vi "Set Property Value.vi"(8 "error in":errorcluster, 10 "Property Type":T1, 11 "Property Type Node":refnum<k20>) -> (0 "error out":errorcluster, 2 "Property Value":variant, 3 "Property Type Node":refnum<k20>)   [LabVIEW 2024, in "Config File Parser.lvlib" / "Property.lvclass"]
uses:
  Property.lvclass
  Property Type.ctl
  DependentFile.ctl
  <vilib>/xml/Close Reference(Node).vi
  Property.lvclass/Property.ctl
  <resource>/objmgr/DOMUserDefRef.rc
  <vilib>/xml/NI_XML.lvlib
  Config File Parser.lvlib
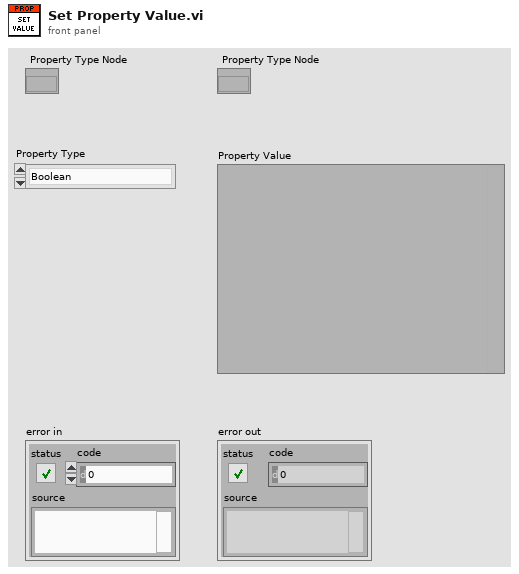
[diagram p1: front panel]
types:
  T1 = typedef "Config File Parser.lvlib/Property.lvclass/Property Type.ctl" = enum16{"Boolean", "Double", "String", "Path", "Dictionary", "DependentFile", "I16", "I32", "I64", "U16", "U32", "U64", "BooleanArray", "DoubleArray", "StringArray", "I16Array", "I32Array", "I64Array", "U16Array", "U32Array", "U64Array", "Variant"}
  T2 = typedef "Config File Parser.lvlib/Property.lvclass/DependentFile.ctl" = cluster{"Path":path, "Version":string, "RTDestination":path, "ForceDownload":bool, "SupportedTarget":string, "MD5":string, " Type":string}
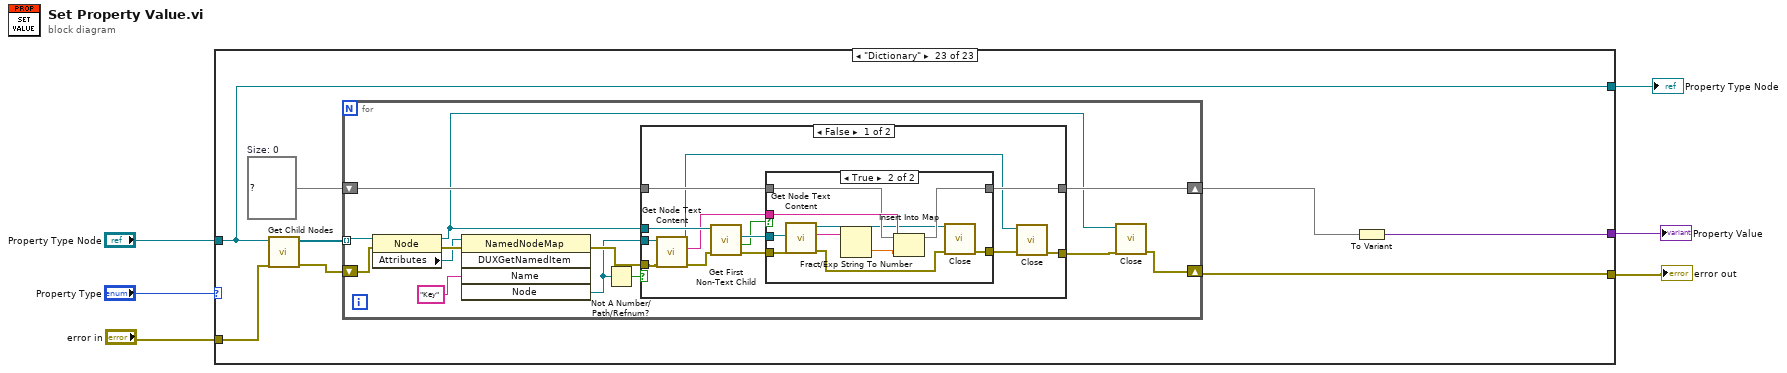
[diagram p0: block diagram]
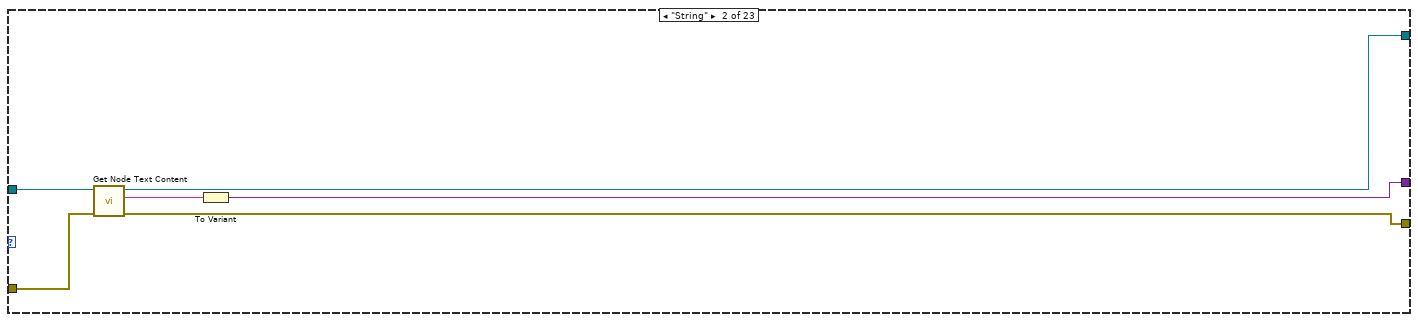
[diagram p3: hidden frame]
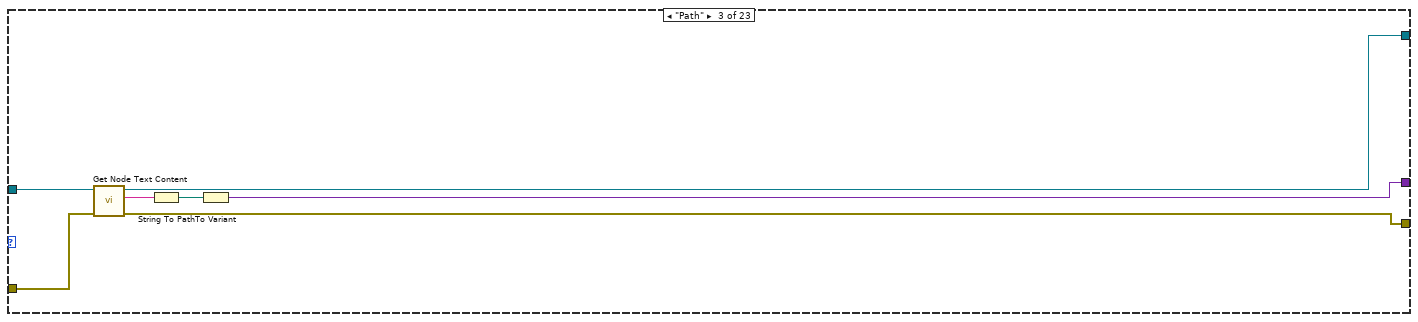
[diagram p4: hidden frame]
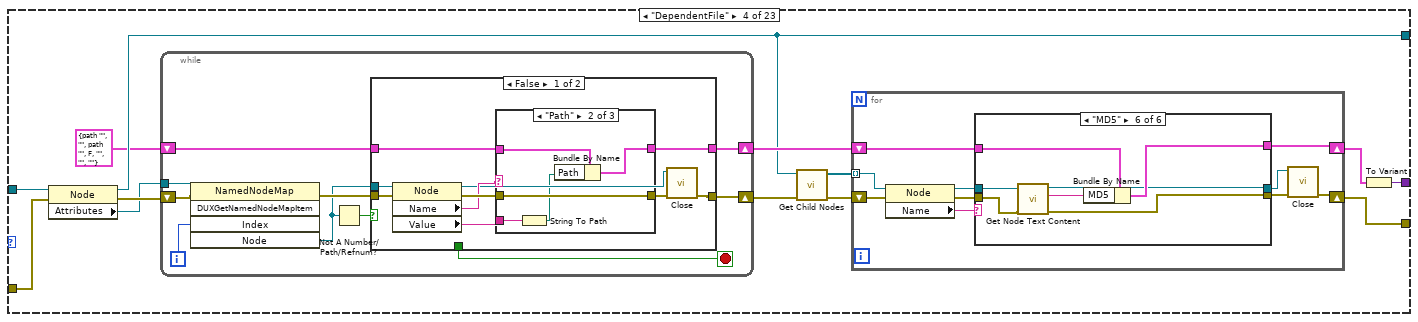
[diagram p5: hidden frame]
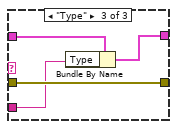
[diagram p7: hidden frame]
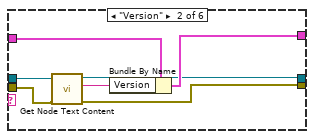
[diagram p10: hidden frame]
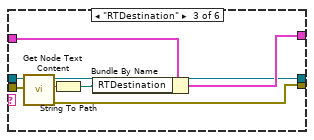
[diagram p11: hidden frame]
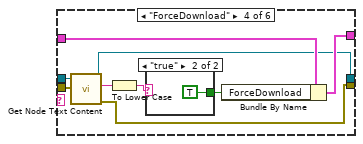
[diagram p12: hidden frame]
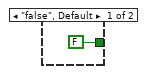
[diagram p13: hidden frame]
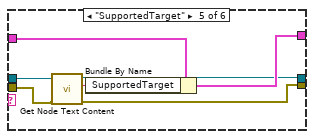
[diagram p14: hidden frame]
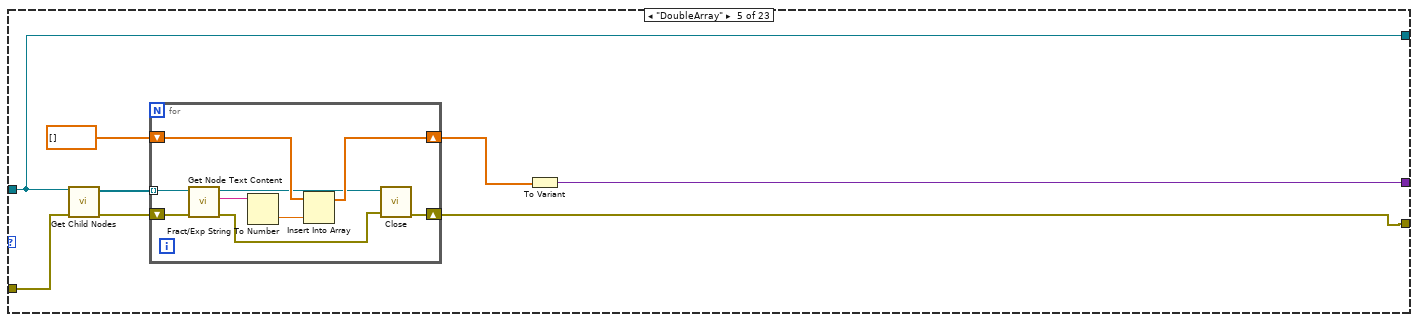
[diagram p15: hidden frame]
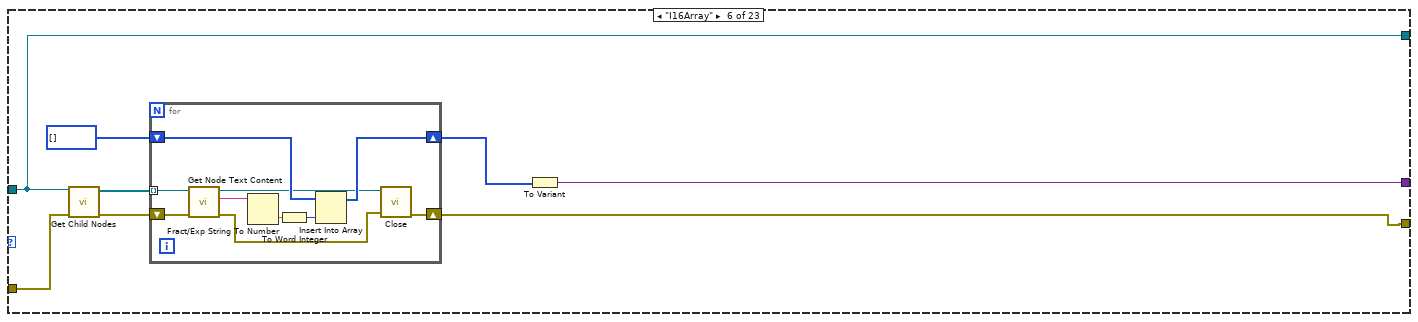
[diagram p16: hidden frame]
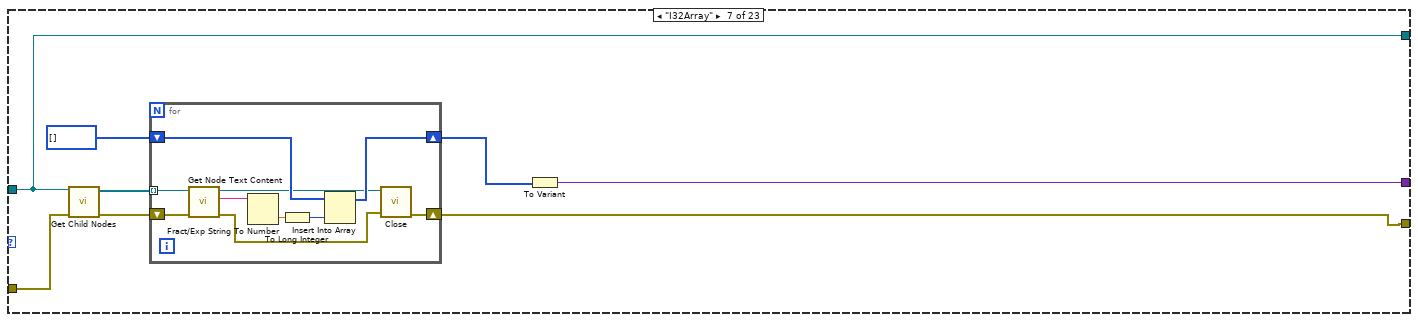
[diagram p17: hidden frame]
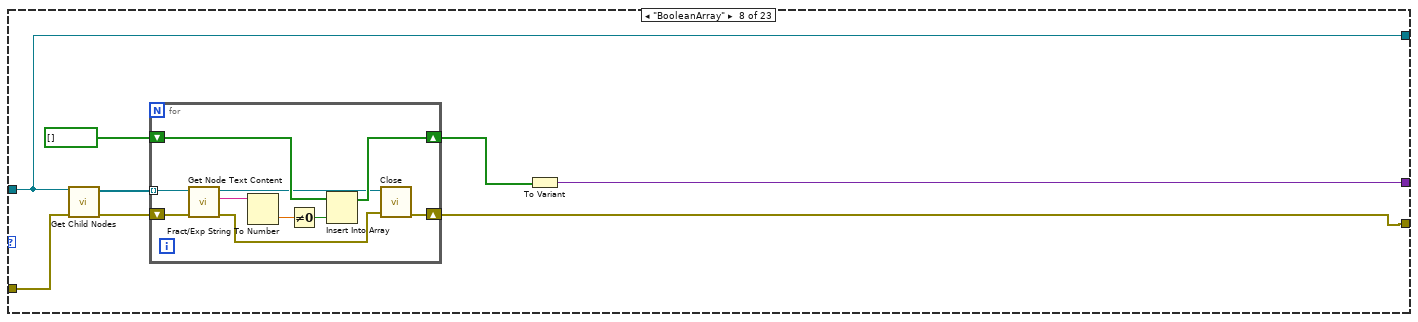
[diagram p18: hidden frame]
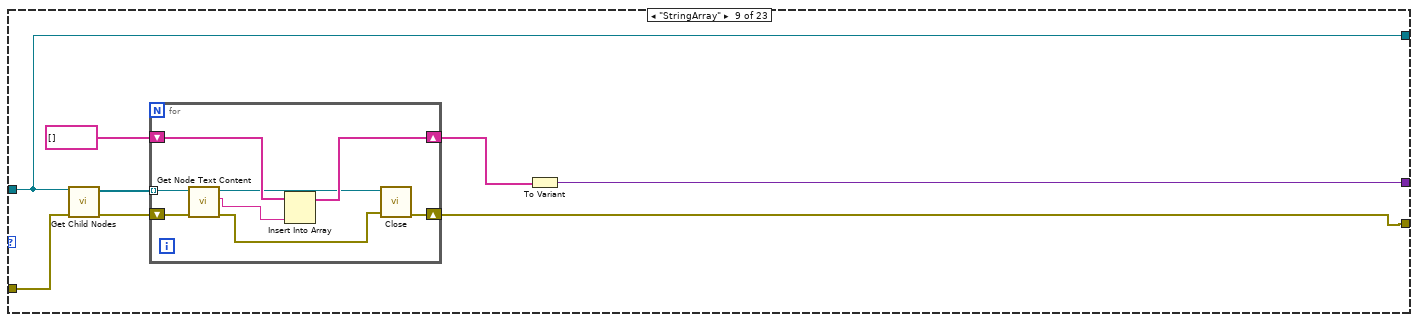
[diagram p19: hidden frame]
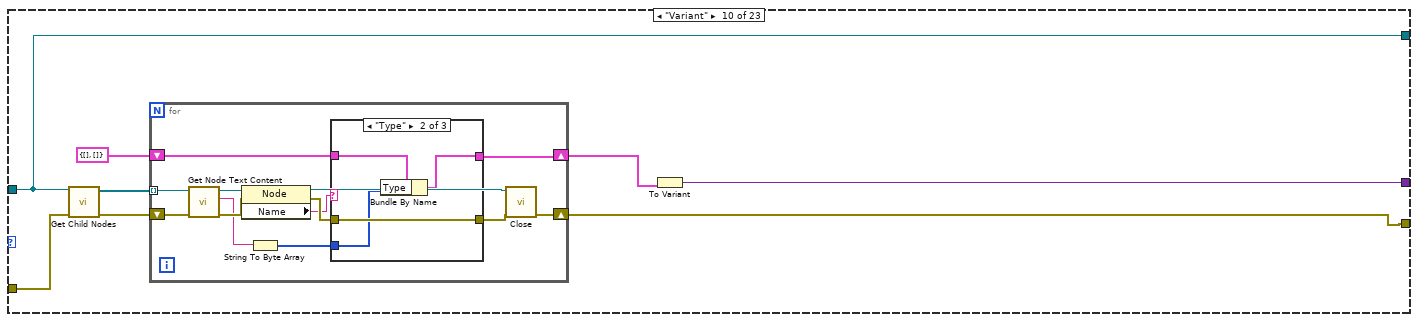
[diagram p20: hidden frame]
diagram:
  n1 = case shown="\"Dictionary\"" "Property Type" {
    tunnel: "Property Type Node" -> [w7 w10 w18 w29 w122 w139 w157 w175 w193 w210 w240 w258 w276 w294 w317 w325 w333 w341 w349 w357 w365 w372 w375]
    tunnel: [_ w12 w19 w27 w124 w141 w159 w177 w195 w212 w242 w260 w278 w296 w312 w320 w328 w336 w344 w352 w362 w369 w377] -> w3
    tunnel: "error in" -> [w8 w14 w21 w34 w128 w145 w163 w181 w199 w215 w246 w264 w282 w300 w319 w327 w335 w343 w351 w359 w367 w374 w382]
    tunnel: [w8 w13 w20 w30 w129 w146 w164 w182 w200 w216 w247 w265 w283 w301 w318 w326 w334 w342 w350 w358 w366 w373 w380] -> w5
    tunnel: [w7 w9 w17 w23 w122 w139 w157 w175 w193 w210 w240 w258 w276 w294 w316 w324 w332 w340 w348 w356 w364 w371 w375] -> w2
    frame Default {
    }
    frame "String" {
      n2 = call <vilib>:"Get Node Text Content.vi"("error in (no error)"=w14, "node in"=w10) -> ("error out"=w13:errorcluster, "node text"=w11:string, "node out"=w9:refnum<k20>)  [unwired: 7 in]
      n3 = To Variant(anything=w11) -> (Variant=w12:variant)
    }
    frame "Path" {
      n4 = call <vilib>:"Get Node Text Content.vi"("error in (no error)"=w21, "node in"=w18) -> ("error out"=w20:errorcluster, "node text"=w16:string, "node out"=w17:refnum<k20>)  [unwired: 7 in]
      n5 = String To Path(string=w16) -> (path=w15:path)
      n6 = To Variant(anything=w15) -> (Variant=w19:variant)
    }
    frame "DependentFile" {
      n7 = property on="Property Node" class="Node"(reference=w29, error in=w34) -> (reference out=w23:refnum<k20>, error out=w33:errorcluster, "Attributes"=w26:refnum<k20>)
      n8 = while {
        tunnel: w26 -> [w41]
        shift-right: [w42] -> w32
        shift-left: w33 -> [w44]
        shift-right: [w35] -> w25
        shift-left: T2 {"Path"=path "", "Version"="", "RTDestination"=path "", "ForceDownload"=FALSE, "SupportedTarget"="", "MD5"="", " Type"=""} ("DependentFile") -> [w36]
        i -> [w40]
        stop <- w37 stop-if-true
        n9 = invoke on="Invoke Node" class="NamedNodeMap" method="DUXGetNamedNodeMapItem"(reference=w41, error in=w44, "Index"=w40) -> (error out=w43:errorcluster, "Node"=w39:refnum<k20>)  [unwired: 2 in, 3 out]
        n10 = Not A Number/Path/Refnum?(number/path/refnum=w39) -> (NaN/Path/Refnum?=w38:bool)
        n11 = case shown="False" w38 {
          selector: w38 -> [_ w67]
          tunnel: w43 -> [w54 w68]
          tunnel: [w46 w68] -> w42
          tunnel: w39 -> [w52 _]
          tunnel: [_ w67] -> w37
          tunnel: w36 -> [w50 w66]
          tunnel: [w48 w66] -> w35
          frame False {
            n12 = property on="Property Node" class="Node"(reference=w52, error in=w54) -> (reference out=w45:refnum<k20>, error out=w53:errorcluster, "Name"=w51:string, "Value"=w49:string)
            n13 = case shown="\"Path\"" w51 {
              tunnel: w50 -> [w55 w60 w64]
              tunnel: w49 -> [_ w59 w63]
              tunnel: [w55 w58 w62] -> w48
              tunnel: w53 -> [w56 w61 w65]
              tunnel: [w56 w61 w65] -> w47
              frame "-1", Default {
              }
              frame "Path" {
                n14 = String To Path(string=w59) -> (path=w57:path)
                n15 = Bundle By Name(cluster=w60, "Path"=w57) -> (w58:T2)
              }
              frame "Type" {
                n16 = Bundle By Name(cluster=w64, "Type"=w63) -> (w62:T2)
              }
            }
            n17 = call-poly <vilib>:"Close.vi"("error in (no error)"=w47, "node"=w45) -> ("error out"=w46:errorcluster)  [unwired: 7 in]
          }
          frame True {
          }
        }
      }
      n18 = call "Get Child Nodes.vi"("error in"=w32, "Node"=w23) -> ("error out"=w31:errorcluster, "Child Nodes"=w28:refnum<k20>[])  [unwired: 8 in]
      n19 = for {
        tunnel: w28 -> [w76] mode=indexing
        shift-right: [w70] -> w30
        shift-left: w31 -> [w78]
        shift-right: [w72] -> w24
        shift-left: w25 -> [w74]
        n20 = property on="Property Node" class="Node"(reference=w76, error in=w78) -> (reference out=w73:refnum<k20>, error out=w77:errorcluster, "Name"=w75:string)
        n21 = case shown="\"MD5\"" w75 {
          tunnel: w74 -> [w80 w86 w94 w104 w112 w119]
          tunnel: w73 -> [w79 w85 w93 w103 w111 w118]
          tunnel: [w80 w83 w91 w102 w109 w116] -> w72
          tunnel: w77 -> [w81 w88 w96 w105 w114 w121]
          tunnel: [w81 w87 w95 w97 w113 w120] -> w71
          tunnel: [w79 w82 w90 w101 w108 w115] -> w69
          frame "-1", Default {
          }
          frame "Version" {
            n22 = call <vilib>:"Get Node Text Content.vi"("error in (no error)"=w88, "node in"=w85) -> ("error out"=w87:errorcluster, "node text"=w84:string, "node out"=w82:refnum<k20>)  [unwired: 7 in]
            n23 = Bundle By Name(cluster=w86, "Version"=w84) -> (w83:T2)
          }
          frame "RTDestination" {
            n24 = call <vilib>:"Get Node Text Content.vi"("error in (no error)"=w96, "node in"=w93) -> ("error out"=w95:errorcluster, "node text"=w92:string, "node out"=w90:refnum<k20>)  [unwired: 7 in]
            n25 = String To Path(string=w92) -> (path=w89:path)
            n26 = Bundle By Name(cluster=w94, "RTDestination"=w89) -> (w91:T2)
          }
          frame "ForceDownload" {
            n27 = call <vilib>:"Get Node Text Content.vi"("error in (no error)"=w105, "node in"=w103) -> ("error out"=w97:errorcluster, "node text"=w100:string, "node out"=w101:refnum<k20>)  [unwired: 7 in]
            n28 = To Lower Case(string=w100) -> (all lower case string=w99:string)
            n29 = case shown="\"true\"" w99 {
              tunnel: [FALSE ("ForceDownload") TRUE ("ForceDownload")] -> w98
              frame "false", Default {
              }
              frame "true" {
              }
            }
            n30 = Bundle By Name(cluster=w104, "ForceDownload"=w98) -> (w102:T2)
          }
          frame "SupportedTarget" {
            n31 = call <vilib>:"Get Node Text Content.vi"("error in (no error)"=w114, "node in"=w111) -> ("error out"=w113:errorcluster, "node text"=w110:string, "node out"=w108:refnum<k20>)  [unwired: 7 in]
            n32 = Bundle By Name(cluster=w112, "SupportedTarget"=w110) -> (w109:T2)
          }
          frame "MD5" {
            n33 = call <vilib>:"Get Node Text Content.vi"("error in (no error)"=w121, "node in"=w118) -> ("error out"=w120:errorcluster, "node text"=w117:string, "node out"=w115:refnum<k20>)  [unwired: 7 in]
            n34 = Bundle By Name(cluster=w119, "MD5"=w117) -> (w116:T2)
          }
        }
        n35 = call-poly <vilib>:"Close.vi"("error in (no error)"=w71, "node"=w69) -> ("error out"=w70:errorcluster)  [unwired: 7 in]
      }
      n36 = To Variant(anything=w24) -> (Variant=w27:variant)
    }
    frame "DoubleArray" {
      n37 = call "Get Child Nodes.vi"("error in"=w128, "Node"=w122) -> ("error out"=w127:errorcluster, "Child Nodes"=w126:refnum<k20>[])  [unwired: 8 in]
      n38 = for {
        tunnel: w126 -> [w135] mode=indexing
        shift-right: [w131] -> w123
        shift-left: dbl[] [] -> [w132]
        shift-right: [w136] -> w129
        shift-left: w127 -> [w138]
        n39 = call <vilib>:"Get Node Text Content.vi"("error in (no error)"=w138, "node in"=w135) -> ("error out"=w137:errorcluster, "node text"=w134:string, "node out"=w130:refnum<k20>)  [unwired: 7 in]
        n40 = Fract/Exp String To Number(string=w134) -> (number=w133:dbl)  [unwired: 3 in, 1 out]
        n41 = Insert Into Array(array=w132, new element=w133) -> (w131:dbl[])  [unwired: 1 in]
        n42 = call-poly <vilib>:"Close.vi"("error in (no error)"=w137, "node"=w130) -> ("error out"=w136:errorcluster)  [unwired: 7 in]
      }
      n43 = To Variant(anything=w123) -> (Variant=w124:variant)
    }
    frame "I16Array" {
      n44 = call "Get Child Nodes.vi"("error in"=w145, "Node"=w139) -> ("error out"=w144:errorcluster, "Child Nodes"=w143:refnum<k20>[])  [unwired: 8 in]
      n45 = for {
        tunnel: w143 -> [w153] mode=indexing
        shift-right: [w149] -> w140
        shift-left: i16[] [] -> [w150]
        shift-right: [w154] -> w146
        shift-left: w144 -> [w156]
        n46 = call <vilib>:"Get Node Text Content.vi"("error in (no error)"=w156, "node in"=w153) -> ("error out"=w155:errorcluster, "node text"=w152:string, "node out"=w148:refnum<k20>)  [unwired: 7 in]
        n47 = Fract/Exp String To Number(string=w152) -> (number=w151:dbl)  [unwired: 3 in, 1 out]
        n48 = To Word Integer(number=w151) -> (16bit integer=w147:i16)
        n49 = Insert Into Array(array=w150, new element=w147) -> (w149:i16[])  [unwired: 1 in]
        n50 = call-poly <vilib>:"Close.vi"("error in (no error)"=w155, "node"=w148) -> ("error out"=w154:errorcluster)  [unwired: 7 in]
      }
      n51 = To Variant(anything=w140) -> (Variant=w141:variant)
    }
    frame "I32Array" {
      n52 = call "Get Child Nodes.vi"("error in"=w163, "Node"=w157) -> ("error out"=w162:errorcluster, "Child Nodes"=w161:refnum<k20>[])  [unwired: 8 in]
      n53 = for {
        tunnel: w161 -> [w171] mode=indexing
        shift-right: [w167] -> w158
        shift-left: i32[] [] -> [w168]
        shift-right: [w172] -> w164
        shift-left: w162 -> [w174]
        n54 = call <vilib>:"Get Node Text Content.vi"("error in (no error)"=w174, "node in"=w171) -> ("error out"=w173:errorcluster, "node text"=w170:string, "node out"=w166:refnum<k20>)  [unwired: 7 in]
        n55 = Fract/Exp String To Number(string=w170) -> (number=w169:dbl)  [unwired: 3 in, 1 out]
        n56 = To Long Integer(number=w169) -> (32bit integer=w165:i32)
        n57 = Insert Into Array(array=w168, new element=w165) -> (w167:i32[])  [unwired: 1 in]
        n58 = call-poly <vilib>:"Close.vi"("error in (no error)"=w173, "node"=w166) -> ("error out"=w172:errorcluster)  [unwired: 7 in]
      }
      n59 = To Variant(anything=w158) -> (Variant=w159:variant)
    }
    frame "BooleanArray" {
      n60 = call "Get Child Nodes.vi"("error in"=w181, "Node"=w175) -> ("error out"=w180:errorcluster, "Child Nodes"=w179:refnum<k20>[])  [unwired: 8 in]
      n61 = for {
        tunnel: w179 -> [w189] mode=indexing
        shift-right: [w185] -> w176
        shift-left: bool[] [] -> [w186]
        shift-right: [w190] -> w182
        shift-left: w180 -> [w192]
        n62 = call <vilib>:"Get Node Text Content.vi"("error in (no error)"=w192, "node in"=w189) -> ("error out"=w191:errorcluster, "node text"=w188:string, "node out"=w184:refnum<k20>)  [unwired: 7 in]
        n63 = Fract/Exp String To Number(string=w188) -> (number=w187:dbl)  [unwired: 3 in, 1 out]
        n64 = Not Equal To 0?(x=w187) -> (x != 0?=w183:bool)
        n65 = Insert Into Array(array=w186, new element=w183) -> (w185:bool[])  [unwired: 1 in]
        n66 = call-poly <vilib>:"Close.vi"("error in (no error)"=w191, "node"=w184) -> ("error out"=w190:errorcluster)  [unwired: 7 in]
      }
      n67 = To Variant(anything=w176) -> (Variant=w177:variant)
    }
    frame "StringArray" {
      n68 = call "Get Child Nodes.vi"("error in"=w199, "Node"=w193) -> ("error out"=w198:errorcluster, "Child Nodes"=w197:refnum<k20>[])  [unwired: 8 in]
      n69 = for {
        tunnel: w197 -> [w205] mode=indexing
        shift-right: [w203] -> w194
        shift-left: string[] [] -> [w204]
        shift-right: [w206] -> w200
        shift-left: w198 -> [w208]
        n70 = call <vilib>:"Get Node Text Content.vi"("error in (no error)"=w208, "node in"=w205) -> ("error out"=w207:errorcluster, "node text"=w201:string, "node out"=w202:refnum<k20>)  [unwired: 7 in]
        n71 = Insert Into Array(array=w204, new element=w201) -> (w203:string[])  [unwired: 1 in]
        n72 = call-poly <vilib>:"Close.vi"("error in (no error)"=w207, "node"=w202) -> ("error out"=w206:errorcluster)  [unwired: 7 in]
      }
      n73 = To Variant(anything=w194) -> (Variant=w195:variant)
    }
    frame "Variant" {
      n74 = call "Get Child Nodes.vi"("error in"=w215, "Node"=w210) -> ("error out"=w214:errorcluster, "Child Nodes"=w213:refnum<k20>[])  [unwired: 8 in]
      n75 = for {
        tunnel: w213 -> [w224] mode=indexing
        shift-right: [w217] -> w211
        shift-left: cluster{"Type":u8[], "Data":u8[]} {"Type"=[], "Data"=[]} -> [w221]
        shift-right: [w228] -> w216
        shift-left: w214 -> [w229]
        n76 = call <vilib>:"Get Node Text Content.vi"("error in (no error)"=w229, "node in"=w224) -> ("error out"=w227:errorcluster, "node text"=w219:string, "node out"=w223:refnum<k20>)  [unwired: 7 in]
        n77 = property class="Node"(reference=w223, error in=w227) -> (reference out=w220:refnum<k20>, error out=w226:errorcluster, "Name"=w222:string)
        n78 = String To Byte Array(string=w219) -> (unsigned byte array=w218:u8[])
        n79 = case shown="\"Type\"" w222 {
          tunnel: w221 -> [w230 w234 w238]
          tunnel: w218 -> [_ w233 w237]
          tunnel: [w230 w232 w236] -> w217
          tunnel: w226 -> [w231 w235 w239]
          tunnel: [w231 w235 w239] -> w225
          frame "-1", Default {
          }
          frame "Type" {
            n80 = Bundle By Name(cluster=w234, "Type"=w233) -> (w232:cluster{"Type":u8[], "Data":u8[]})
          }
          frame "Data" {
            n81 = Bundle By Name(cluster=w238, "Data"=w237) -> (w236:cluster{"Type":u8[], "Data":u8[]})
          }
        }
        n82 = call-poly <vilib>:"Close.vi"("error in (no error)"=w225, "node"=w220) -> ("error out"=w228:errorcluster)  [unwired: 7 in]
      }
      n83 = To Variant(anything=w211) -> (Variant=w212:variant)
    }
    frame "I64Array" {
      n84 = call "Get Child Nodes.vi"("error in"=w246, "Node"=w240) -> ("error out"=w245:errorcluster, "Child Nodes"=w244:refnum<k20>[])  [unwired: 8 in]
      n85 = for {
        tunnel: w244 -> [w254] mode=indexing
        shift-right: [w250] -> w241
        shift-left: i64[] [] -> [w251]
        shift-right: [w255] -> w247
        shift-left: w245 -> [w257]
        n86 = call <vilib>:"Get Node Text Content.vi"("error in (no error)"=w257, "node in"=w254) -> ("error out"=w256:errorcluster, "node text"=w253:string, "node out"=w249:refnum<k20>)  [unwired: 7 in]
        n87 = Fract/Exp String To Number(string=w253) -> (number=w252:dbl)  [unwired: 3 in, 1 out]
        n88 = To Quad Integer(1:w252) -> (0:w248:i64)
        n89 = Insert Into Array(array=w251, new element=w248) -> (w250:i64[])  [unwired: 1 in]
        n90 = call-poly <vilib>:"Close.vi"("error in (no error)"=w256, "node"=w249) -> ("error out"=w255:errorcluster)  [unwired: 7 in]
      }
      n91 = To Variant(anything=w241) -> (Variant=w242:variant)
    }
    frame "U16Array" {
      n92 = call "Get Child Nodes.vi"("error in"=w264, "Node"=w258) -> ("error out"=w263:errorcluster, "Child Nodes"=w262:refnum<k20>[])  [unwired: 8 in]
      n93 = for {
        tunnel: w262 -> [w272] mode=indexing
        shift-right: [w268] -> w259
        shift-left: u16[] [] -> [w269]
        shift-right: [w273] -> w265
        shift-left: w263 -> [w275]
        n94 = call <vilib>:"Get Node Text Content.vi"("error in (no error)"=w275, "node in"=w272) -> ("error out"=w274:errorcluster, "node text"=w271:string, "node out"=w267:refnum<k20>)  [unwired: 7 in]
        n95 = Fract/Exp String To Number(string=w271) -> (number=w270:dbl)  [unwired: 3 in, 1 out]
        n96 = To Unsigned Word Integer(number=w270) -> (unsigned 16bit integer=w266:u16)
        n97 = Insert Into Array(array=w269, new element=w266) -> (w268:u16[])  [unwired: 1 in]
        n98 = call-poly <vilib>:"Close.vi"("error in (no error)"=w274, "node"=w267) -> ("error out"=w273:errorcluster)  [unwired: 7 in]
      }
      n99 = To Variant(anything=w259) -> (Variant=w260:variant)
    }
    frame "U32Array" {
      n100 = call "Get Child Nodes.vi"("error in"=w282, "Node"=w276) -> ("error out"=w281:errorcluster, "Child Nodes"=w280:refnum<k20>[])  [unwired: 8 in]
      n101 = for {
        tunnel: w280 -> [w290] mode=indexing
        shift-right: [w286] -> w277
        shift-left: u32[] [] -> [w287]
        shift-right: [w291] -> w283
        shift-left: w281 -> [w293]
        n102 = call <vilib>:"Get Node Text Content.vi"("error in (no error)"=w293, "node in"=w290) -> ("error out"=w292:errorcluster, "node text"=w289:string, "node out"=w285:refnum<k20>)  [unwired: 7 in]
        n103 = Fract/Exp String To Number(string=w289) -> (number=w288:dbl)  [unwired: 3 in, 1 out]
        n104 = To Unsigned Long Integer(number=w288) -> (unsigned 32bit integer=w284:u32)
        n105 = Insert Into Array(array=w287, new element=w284) -> (w286:u32[])  [unwired: 1 in]
        n106 = call-poly <vilib>:"Close.vi"("error in (no error)"=w292, "node"=w285) -> ("error out"=w291:errorcluster)  [unwired: 7 in]
      }
      n107 = To Variant(anything=w277) -> (Variant=w278:variant)
    }
    frame "U64Array" {
      n108 = call "Get Child Nodes.vi"("error in"=w300, "Node"=w294) -> ("error out"=w299:errorcluster, "Child Nodes"=w298:refnum<k20>[])  [unwired: 8 in]
      n109 = for {
        tunnel: w298 -> [w308] mode=indexing
        shift-right: [w304] -> w295
        shift-left: u64[] [] -> [w305]
        shift-right: [w309] -> w301
        shift-left: w299 -> [w311]
        n110 = call <vilib>:"Get Node Text Content.vi"("error in (no error)"=w311, "node in"=w308) -> ("error out"=w310:errorcluster, "node text"=w307:string, "node out"=w303:refnum<k20>)  [unwired: 7 in]
        n111 = Fract/Exp String To Number(string=w307) -> (number=w306:dbl)  [unwired: 3 in, 1 out]
        n112 = To Unsigned Quad Integer(1:w306) -> (0:w302:u64)
        n113 = Insert Into Array(array=w305, new element=w302) -> (w304:u64[])  [unwired: 1 in]
        n114 = call-poly <vilib>:"Close.vi"("error in (no error)"=w310, "node"=w303) -> ("error out"=w309:errorcluster)  [unwired: 7 in]
      }
      n115 = To Variant(anything=w295) -> (Variant=w296:variant)
    }
    frame "U32" {
      n116 = call <vilib>:"Get Node Text Content.vi"("error in (no error)"=w319, "node in"=w317) -> ("error out"=w318:errorcluster, "node text"=w315:string, "node out"=w316:refnum<k20>)  [unwired: 7 in]
      n117 = Fract/Exp String To Number(string=w315) -> (number=w314:dbl)  [unwired: 3 in, 1 out]
      n118 = To Unsigned Long Integer(number=w314) -> (unsigned 32bit integer=w313:u32)
      n119 = To Variant(anything=w313) -> (Variant=w312:variant)
    }
    frame "U16" {
      n120 = call <vilib>:"Get Node Text Content.vi"("error in (no error)"=w327, "node in"=w325) -> ("error out"=w326:errorcluster, "node text"=w323:string, "node out"=w324:refnum<k20>)  [unwired: 7 in]
      n121 = Fract/Exp String To Number(string=w323) -> (number=w322:dbl)  [unwired: 3 in, 1 out]
      n122 = To Unsigned Word Integer(number=w322) -> (unsigned 16bit integer=w321:u16)
      n123 = To Variant(anything=w321) -> (Variant=w320:variant)
    }
    frame "U64" {
      n124 = call <vilib>:"Get Node Text Content.vi"("error in (no error)"=w335, "node in"=w333) -> ("error out"=w334:errorcluster, "node text"=w331:string, "node out"=w332:refnum<k20>)  [unwired: 7 in]
      n125 = Fract/Exp String To Number(string=w331) -> (number=w330:dbl)  [unwired: 3 in, 1 out]
      n126 = To Unsigned Quad Integer(1:w330) -> (0:w329:u64)
      n127 = To Variant(anything=w329) -> (Variant=w328:variant)
    }
    frame "I16" {
      n128 = call <vilib>:"Get Node Text Content.vi"("error in (no error)"=w343, "node in"=w341) -> ("error out"=w342:errorcluster, "node text"=w339:string, "node out"=w340:refnum<k20>)  [unwired: 7 in]
      n129 = Fract/Exp String To Number(string=w339) -> (number=w338:dbl)  [unwired: 3 in, 1 out]
      n130 = To Word Integer(number=w338) -> (16bit integer=w337:i16)
      n131 = To Variant(anything=w337) -> (Variant=w336:variant)
    }
    frame "I32" {
      n132 = call <vilib>:"Get Node Text Content.vi"("error in (no error)"=w351, "node in"=w349) -> ("error out"=w350:errorcluster, "node text"=w347:string, "node out"=w348:refnum<k20>)  [unwired: 7 in]
      n133 = Fract/Exp String To Number(string=w347) -> (number=w346:dbl)  [unwired: 3 in, 1 out]
      n134 = To Long Integer(number=w346) -> (32bit integer=w345:i32)
      n135 = To Variant(anything=w345) -> (Variant=w344:variant)
    }
    frame "I64" {
      n136 = call <vilib>:"Get Node Text Content.vi"("error in (no error)"=w359, "node in"=w357) -> ("error out"=w358:errorcluster, "node text"=w355:string, "node out"=w356:refnum<k20>)  [unwired: 7 in]
      n137 = Fract/Exp String To Number(string=w355) -> (number=w354:dbl)  [unwired: 3 in, 1 out]
      n138 = To Quad Integer(1:w354) -> (0:w353:i64)
      n139 = To Variant(anything=w353) -> (Variant=w352:variant)
    }
    frame "Boolean" {
      n140 = call <vilib>:"Get Node Text Content.vi"("error in (no error)"=w367, "node in"=w365) -> ("error out"=w366:errorcluster, "node text"=w363:string, "node out"=w364:refnum<k20>)  [unwired: 7 in]
      n141 = Fract/Exp String To Number(string=w363) -> (number=w360:dbl)  [unwired: 3 in, 1 out]
      n142 = Not Equal To 0?(x=w360) -> (x != 0?=w361:bool)
      n143 = To Variant(anything=w361) -> (Variant=w362:variant)
    }
    frame "Double" {
      n144 = call <vilib>:"Get Node Text Content.vi"("error in (no error)"=w374, "node in"=w372) -> ("error out"=w373:errorcluster, "node text"=w370:string, "node out"=w371:refnum<k20>)  [unwired: 7 in]
      n145 = Fract/Exp String To Number(string=w370) -> (number=w368:dbl)  [unwired: 3 in, 1 out]
      n146 = To Variant(anything=w368) -> (Variant=w369:variant)
    }
    frame "Dictionary" {
      w379 = map{string, dbl} {}  # Size: 0
      n147 = call "Get Child Nodes.vi"("error in"=w382, "Node"=w375) -> ("error out"=w381:errorcluster, "Child Nodes"=w378:refnum<k20>[])  [unwired: 8 in]
      n148 = for {
        shift-right: [w388] -> w376
        shift-left: w379 -> [w389]
        tunnel: w378 -> [w387] mode=indexing
        shift-right: [w391] -> w380
        shift-left: w381 -> [w394]
        n149 = property on="Property Node" class="Node"(reference=w387, error in=w394) -> (reference out=w383:refnum<k20>, error out=w395:errorcluster, "Attributes"=w390:refnum<k20>)
        n150 = invoke on="Invoke Node" class="NamedNodeMap" method="DUXGetNamedItem"(reference=w390, error in=w395, "Name"="Key") -> (error out=w393:errorcluster, "Node"=w385:refnum<k20>)  [unwired: 2 in, 3 out]
        n151 = Not A Number/Path/Refnum?(number/path/refnum=w385) -> (NaN/Path/Refnum?=w384:bool)
        n152 = case shown="False" w384 {
          tunnel: w385 -> [w403 _]
          tunnel: w383 -> [w402 _]
          tunnel: w389 -> [w400 w421]
          tunnel: [w399 w421] -> w388
          tunnel: w393 -> [w407 w422]
          tunnel: [w404 w422] -> w392
          frame False {
            n153 = call <vilib>:"Get Node Text Content.vi"("error in (no error)"=w407, "node in"=w403) -> ("error out"=w406:errorcluster, "node text"=w401:string, "node out"=w397:refnum<k20>)  [unwired: 7 in]
            n154 = call <vilib>:"Get First Non-Text Child.vi"("error in (no error)"=w406, "node in"=w402) -> ("error out"=w408:errorcluster, "found child node?"=w396:bool, "child node"=w398:refnum<k20>)  [unwired: 6 in, 1 out]
            n155 = case shown="True" w396 {
              tunnel: w408 -> [w410 w420]
              tunnel: w401 -> [_ w417]
              tunnel: w400 -> [w409 w416]
              tunnel: [w409 w415] -> w399
              tunnel: w398 -> [_ w414]
              tunnel: [w410 w418] -> w405
              frame False {
              }
              frame True {
                n156 = call <vilib>:"Get Node Text Content.vi"("error in (no error)"=w420, "node in"=w414) -> ("error out"=w419:errorcluster, "node text"=w412:string, "node out"=w413:refnum<k20>)  [unwired: 7 in]
                n157 = Fract/Exp String To Number(string=w412) -> (number=w411:dbl)  [unwired: 3 in, 1 out]
                n158 = Insert Into Map(map in=w416, key=w417, value=w411) -> (map out=w415:map{string, dbl})  [unwired: 2 out]
                n159 = call-poly <vilib>:"Close.vi"("error in (no error)"=w419, "node"=w413) -> ("error out"=w418:errorcluster)  [unwired: 7 in]
              }
            }
            n160 = call-poly <vilib>:"Close.vi"("error in (no error)"=w405, "node"=w397) -> ("error out"=w404:errorcluster)  [unwired: 7 in]
          }
          frame True {
          }
        }
        n161 = call-poly <vilib>:"Close.vi"("error in (no error)"=w392, "node"=w383) -> ("error out"=w391:errorcluster)  [unwired: 7 in]
      }
      n162 = To Variant(anything=w376) -> (Variant=w377:variant)
    }
  }
  "Property Value" <- w3
  "error out" <- w5
  "Property Type Node" <- w2
